vi "get&set ReadOnly.vi"(6 "Get/Set? (Set)":bool=TRUE, 8 "error in (no error)":errorcluster, 10 "ReadOnly":bool, 11 "VGS_ComponentInfo in":refnum<class "VGS_ComponentInfo.lvclass">) -> (0 "error out":errorcluster, 2 "ReadOnly":bool, 3 "VGS_ComponentInfo out":refnum<class "VGS_ComponentInfo.lvclass">)   [LabVIEW 2022 SP3, in "LV_VGS.lvlib" / "VGS_ComponentInfo.lvclass"]
uses:
  VGS_ComponentInfo.lvclass
  VGS_ComponentInfo.lvclass/VGS_ComponentInfo.ctl
  C:/Users/Andrey/Documents/GitHub/LV_VGS/vgs_project.dll
  vgs_project.dll
panel:
  # "-Set\n-Get"
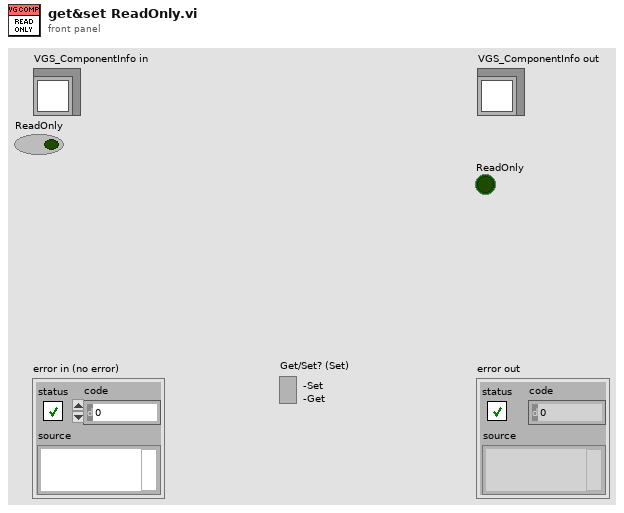
[diagram p1: front panel]
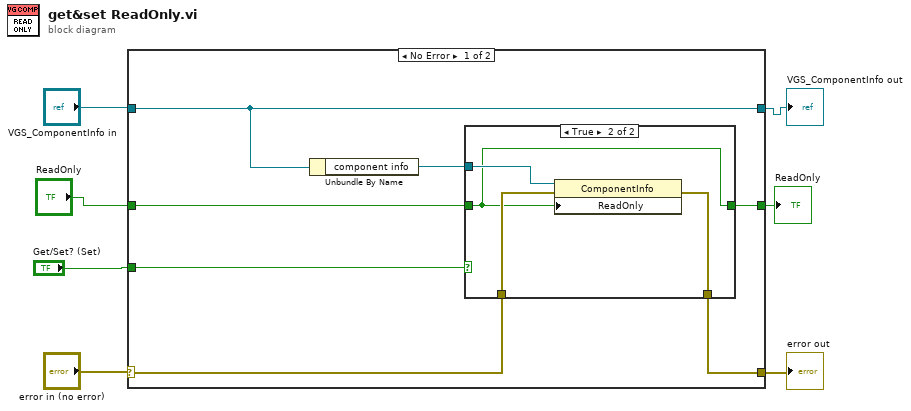
[diagram p0: block diagram]
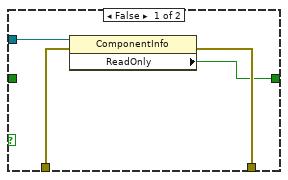
[diagram p2: hidden frame]
diagram:
  n1 = case shown="No Error" "error in (no error)" {
    selector: "error in (no error)" -> [w12 w25]
    tunnel: [w11 w25] -> w5
    tunnel: [w14 w24] -> w6
    tunnel: "VGS_ComponentInfo in" -> [w14 w24]
    tunnel: "Get/Set? (Set)" -> [w10 _]
    tunnel: "ReadOnly" -> [w9 w23]
    tunnel: [w8 w23] -> w2
    frame No Error {
      n2 = Unbundle By Name(w14) -> ("component info"=w13:refnum<k24>)
      n3 = case shown="True" w10 {
        tunnel: w13 -> [w18 w20]
        tunnel: w12 -> [w17 w22]
        tunnel: [w16 w21] -> w11
        tunnel: w9 -> [_ w19]
        tunnel: [w15 w19] -> w8
        frame False {
          n4 = property class="ComponentInfo"(reference=w18, error in=w17) -> (error out=w16:errorcluster, "ReadOnly"=w15:bool)  [unwired: 1 out]
        }
        frame True {
          n5 = property class="ComponentInfo"(reference=w20, error in=w22, "ReadOnly"=w19) -> (error out=w21:errorcluster)  [unwired: 1 out]
        }
      }
    }
    frame Error {
    }
  }
  "error out" <- w5
  "VGS_ComponentInfo out" <- w6
  "ReadOnly" <- w2
